vi "TOSA_MCS_Switch_SA.vi"() -> ()   [LabVIEW 2012]
panel:
  in  "Stop":bool
  in  "TOSA/MCS":bool=TRUE
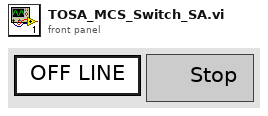
[diagram p1: front panel]
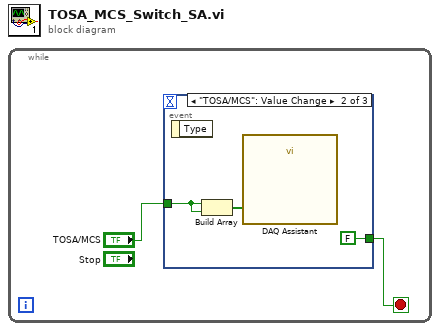
[diagram p0: block diagram]
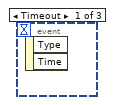
[diagram p2: hidden frame]
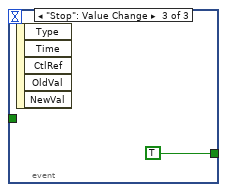
[diagram p3: hidden frame]
diagram:
  n1 = while {
    stop <- w1 stop-if-true
    n2 = event shown="[1] \"TOSA/MCS\": Value Change" {
      selector: _ -> [_ _ _]
      dyn-events: _ -> [_ _ _]
      timeout: _ -> [_ _ _]
      tunnel: "TOSA/MCS" -> [_ w4 _]
      tunnel: [_ FALSE TRUE] -> w1
      event Timeout {
        n3 = event-data() -> ()  [unwired: 1 in, 2 out]
      }
      event "TOSA/MCS": Value Change {
        n4 = event-data() -> ()  [unwired: 1 in, 1 out]
        n5 = Build Array(w4, w4) -> (w5:bool[])
        n6 = call "DAQ Assistant"("data"=w5) -> ()  [unwired: 17 in, 2 out]
      }
      event "Stop": Value Change {
        n7 = event-data() -> ()  [unwired: 1 in, 5 out]
      }
    }
  }
